vi "WPI_SetFilterFrequency.vi"(8 "error in (no error)":errorcluster, 10 "Filter Frequency":dbl=76628.35249042146, 11 "DigitalInputDevRef":T1={"DevStatus"={"status"=FALSE, "code"=0, "source"=""}, "DIO Channel"=enum."DIO 1"}) -> (0 "error out":errorcluster, 3 "DigitalInputDevRef":T1={"DevStatus"={"status"=FALSE, "code"=0, "source"=""}, "DIO Channel"=enum."DIO 1"})   [LabVIEW 2017]
doc: "Enables a digital input filter and configures the filter frequency.\n\nThis software is licensed. Open the labview\\readme\\WPI Robotics Library Open Source License.txt file for more information."
uses:
  <vilib>/Rock Robotics/WPI/DigitalInput/WPI_DigitalInputDevRef.ctl
  <vilib>/Rock Robotics/SystemInterfaces/DIO/FPGA_DIOChannel.ctl
  <vilib>/Rock Robotics/SystemInterfaces/NetworkCommunication/NetComm_UsageReport_ResourceType.ctl
  <vilib>/Rock Robotics/SystemInterfaces/System/FPGA_SystemGet.vi
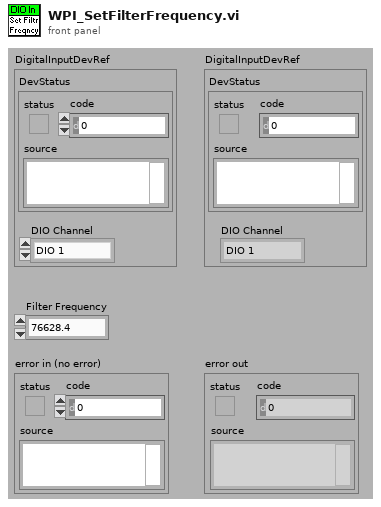
[diagram p1: front panel]
types:
  T1 = typedef "WPI_DigitalInputDevRef.ctl" = cluster{"DevStatus":errorcluster, "DIO Channel":T2}
  T2 = typedef "FPGA_DIOChannel.ctl" = enum8{"DIO 0", "DIO 1", "DIO 2", "DIO 3", "DIO 4", "DIO 5", "DIO 6", "DIO 7", "DIO 8", "DIO 9", "DIO MXP 0", "DIO MXP 1", "DIO MXP 2", "DIO MXP 3", "DIO MXP 4", "DIO MXP 5", "DIO MXP 6", "DIO MXP 7", "DIO MXP 8", "DIO MXP 9", "DIO MXP 10", "DIO MXP 11", "DIO MXP 12", "DIO MXP 13", "DIO MXP 14", "DIO MXP 15", "SPI Port CS1", "SPI Port CS2", "SPI Port CS3", "SPI Port MISO", "SPI Port MOSI", "Invalid"}
  T3 = typedef "NetComm_UsageReport_ResourceType.ctl" = enum8{"Controller", "Module", "Language", "CANPlugin", "Accelerometer", "ADXL345", "AnalogChannel", "AnalogTrigger", "AnalogTriggerOutput", "CANJaguar", "Compressor", "Counter", "Dashboard", "DigitalInput", "DigitalOutput", "DriverStationCIO", "DriverStationEIO", "DriverStationLCD", "Encoder", "GearTooth", "Gyro", "I2C", "Framework", "Jaguar", "Joystick", "Kinect", "KinectStick", "PIDController", "Preferences", "PWM", "Relay", "RobotDrive", "SerialPort", "Servo", "Solenoid", "SPI", "Task", "Ultrasonic", "Victor", "Button", "Command", "AxisCamera", "PCVideoServer", "SmartDashboard", "Talon", "HiTechnicColorSensor", "HiTechnicAccel", "HiTechnicCompass", "SRF08", "AnalogOutput", "Victor SP", "Talon SRX", "CAN Talon SRX", "ADXL362 Accel", "ADXRS450 Gyro", "Rev SPARK", "Mindsensors SD540", "Digital Filter", "ADIS16448", "PDP", "PCM", "PigeonIMU", "Nidec Brushless", "CTRE CANifier", "CTRE Future 0", "CTRE Future 1", "CTRE Future 2", "CTRE Future 3", "CTRE Future 4", "CTRE Future 5", "CTRE Future 6"}
  T4 = typedef "FPGA_DIODevRef.ctl" = cluster{"DevStatus":errorcluster}
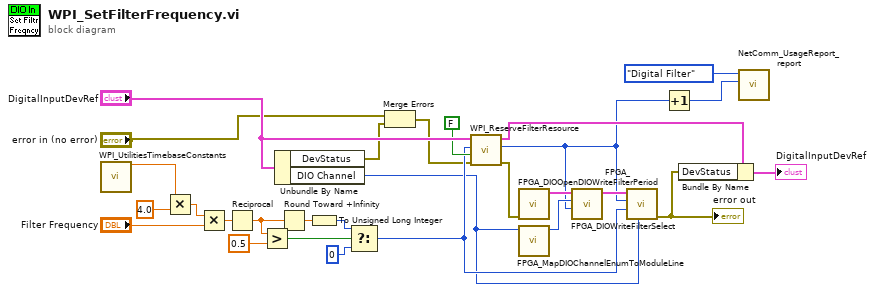
[diagram p0: block diagram]
diagram:
  n1 = call <vilib>:"WPI_UtilitiesTimebaseConstants.vi"() -> ("40 MHz FPGA clock"=w4:dbl)  [unwired: 13 in, 2 out]
  n2 = Multiply(x=w4, y=4.0) -> (x*y=w22:dbl)
  n3 = Multiply(x=w22, y="Filter Frequency") -> (x*y=w23:dbl)
  n4 = Reciprocal(x=w23) -> (1/x=w15:dbl)
  n5 = Greater?(x=w15, y=0.5) -> (0:w19:bool)
  n6 = Unbundle By Name("DigitalInputDevRef") -> ("DevStatus"=w7:errorcluster, "DIO Channel"=w5:T2)
  n7 = Round Toward +Infinity(x=w15) -> (ceil(x): smallest int >= x=w16:dbl)
  n8 = To Unsigned Long Integer(number=w16) -> (unsigned 32bit integer=w18:u32)
  n9 = Select(t=w18, s=w19, f=u32 0) -> (s? t:f=w9:u32)
  n10 = Merge Errors("error in (no error)", w7) -> (w6:errorcluster)
  n11 = call <vilib>:"WPI_ReserveFilterResource.vi"("error in (no error)"=w6, "Release Filter"=FALSE, "Filter Period"=w9, "DigitalInputDevRef"="DigitalInputDevRef") -> ("error out"=w13:errorcluster, "Filter Index"=w1:u8, "DigitalInputDevRef"=w26:T1)  [unwired: 5 out]
  n12 = call <vilib>:"FPGA_DIOOpen.vi"("error in (no error)"=w13) -> ("DIODeviceRef"=w12:T4)  [unwired: 1 in, 9 out]
  n13 = call <vilib>:"FPGA_MapDIOChannelEnumToModuleLine.vi"("DIOChannel"=w5) -> ("ActualDIOChannel(U8)"=w11:u8)  [unwired: 10 out]
  n14 = call <vilib>:"FPGA_DIOWriteFilterSelect.vi"("PWMFilterSelect"=w1, "channel index"=w11, "DIODeviceRef"=w12) -> ("DIODeviceRef"=w10:T4)  [unwired: 1 in, 7 out]
  n15 = call <vilib>:"FPGA_DIOWriteFilterPeriod.vi"("DIOChannel"=w5, "PWMFilterPeriod"=w9, "filter index"=w1, "DIODeviceRef In"=w10) -> ("error out"=w24:errorcluster)  [unwired: 1 in, 6 out]
  "error out" <- w24
  n16 = Increment(x=w1) -> (x+1=w2:u8)
  n17 = Bundle By Name(cluster=w26, "DevStatus"=w24) -> (→"DigitalInputDevRef":T1)
  n18 = call <vilib>:"NetComm_UsageReport_report.vi"("Instance Number"=w2, "Resource Type"=NetComm_UsageReport_ResourceType."Digital Filter") -> ()  [unwired: 10 in]
